vi "Do.vi"(8 "error in (no error)":errorcluster, 10 "DMM":refnum<class "DMM.lvclass">, 11 "Reset DMM in":refnum<class "Reset DMM.lvclass">) -> (0 "error out":errorcluster, 2 "DMM":refnum<class "DMM.lvclass">, 3 "Reset DMM out":refnum<class "Reset DMM.lvclass">)   [LabVIEW 2020, in "Reset DMM.lvclass"]
uses:
  Reset DMM.lvclass
  DMM/DMM.lvclass
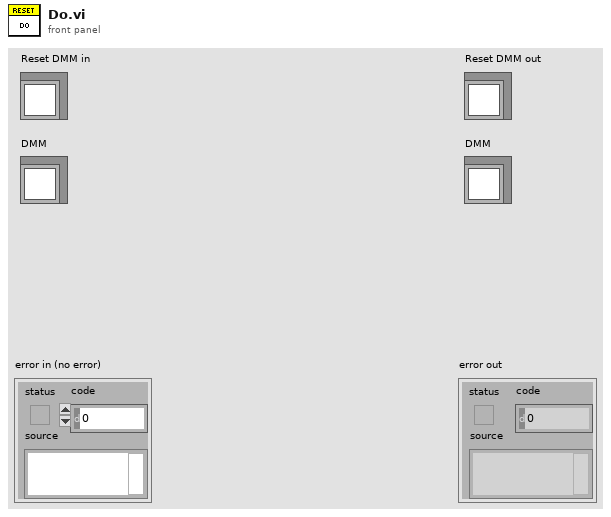
[diagram p1: front panel]
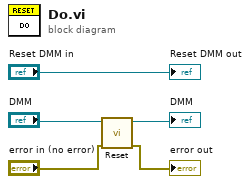
[diagram p0: block diagram]
diagram:
  n1 = call-dynamic "Reset.vi"("error in (no error)"="error in (no error)", "DMM in"="DMM") -> ("error out"=→"error out":errorcluster, "DMM out"=→"DMM":refnum<class "DMM.lvclass">)  [unwired: 8 in]
  "Reset DMM out" <- "Reset DMM in"
